vi "Frame (ms) Write.vi"(4 "error in (no error)":errorcluster, 5 "Value":dbl, 6 "Container State":T5, 7 "Display State In":T1) -> (0 "error out":errorcluster, 3 "Display State Out":T1)   [LabVIEW 2020, in "SignalManager.xctl"]
uses:
  SignalManager.xctl
  <vilib>/_xctls/Container State.ctl
  <vilib>/_xctls/XControlSupport.lvlib
  Event Data.ctl
  Events.ctl
  Utility VIs/Controls/KListboxEx/Event Action.ctl
  Utility VIs/Controls/KListboxEx/KListboxEx.xctl
  Utility VIs/Controls/KListboxEx/Events.ctl
  PeriodDisplay.ctl
  State.ctl
panel:
  # "Replace the Value Control below with a Control of desired type.\nDo not remove this Control or the others from the connector pane.\nDo not change the connector pane pattern.\nThe Value control should always be the third terminal from top on the input side in the connector pane."
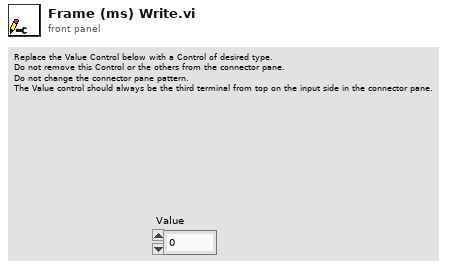
[diagram p1: front panel]
types:
  T1 = typedef "SignalManager.xctl/State.ctl" = cluster{"Channels":T2, "Destinations":string[], "action":string, "EventReg":refnum<event-registration>, "selectedChan":i32, "Period Display":T3, "Events":T4, "Fs (Hz)":dbl, "TDT":bool, "Frame (ms)":dbl}
  T2 = typedef "KListboxEx.xctl/Events.ctl" = cluster{"Items Changed":refnum<user-event>, "List Changed":refnum<user-event>}
  T3 = typedef "SignalManager.xctl/PeriodDisplay.ctl" = enum16{"Interval", "RepRate", "Both"}
  T4 = typedef "SignalManager.xctl/Events.ctl" = cluster{"Rename":refnum<user-event>}
  T5 = typedef "XControlSupport.lvlib/Container State.ctl" = cluster{"Indicator?":bool, "Run Mode?":bool, " Refnum":refnum<vi>}
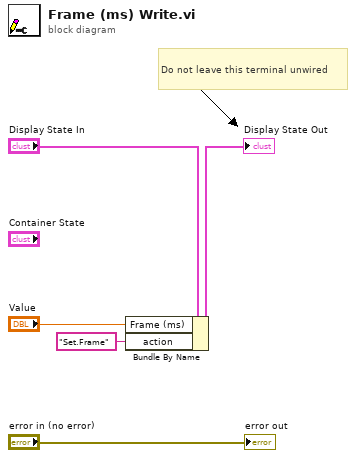
[diagram p0: block diagram]
diagram:
  # "Do not leave this terminal unwired"
  n1 = Bundle By Name(cluster="Display State In", "Frame (ms)"="Value", "action"="Set.Frame") -> (→"Display State Out":T1)
  "error out" <- "error in (no error)"
